vi "Launch Test Bench.vi"(4 "Monitor":enum16{"Primary", "1", "2", "3"}(ring), 6 "Station":T1(ring), 7 "wait until completion? (F)":bool, 8 "error in (no error)":errorcluster, 11 "App Path":path) -> (0 "error out":errorcluster)   [LabVIEW 2019, in "Test Bench Tools.lvlib"]
uses:
  Test Bench Tools.lvlib
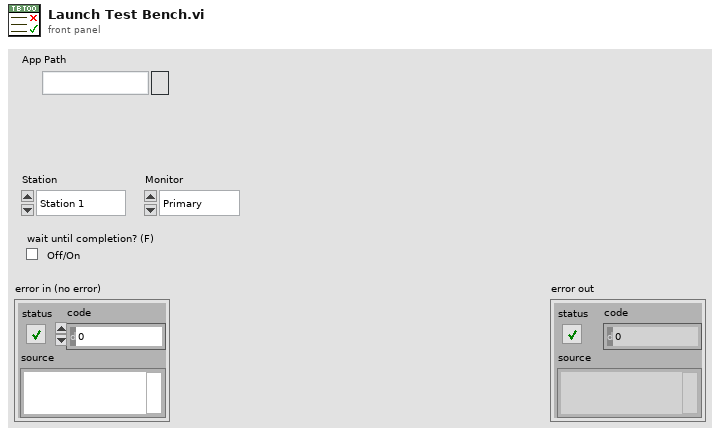
[diagram p1: front panel]
types:
  T1 = enum16{"Station 1", "Station 2", "Station 3", "Station 4"}
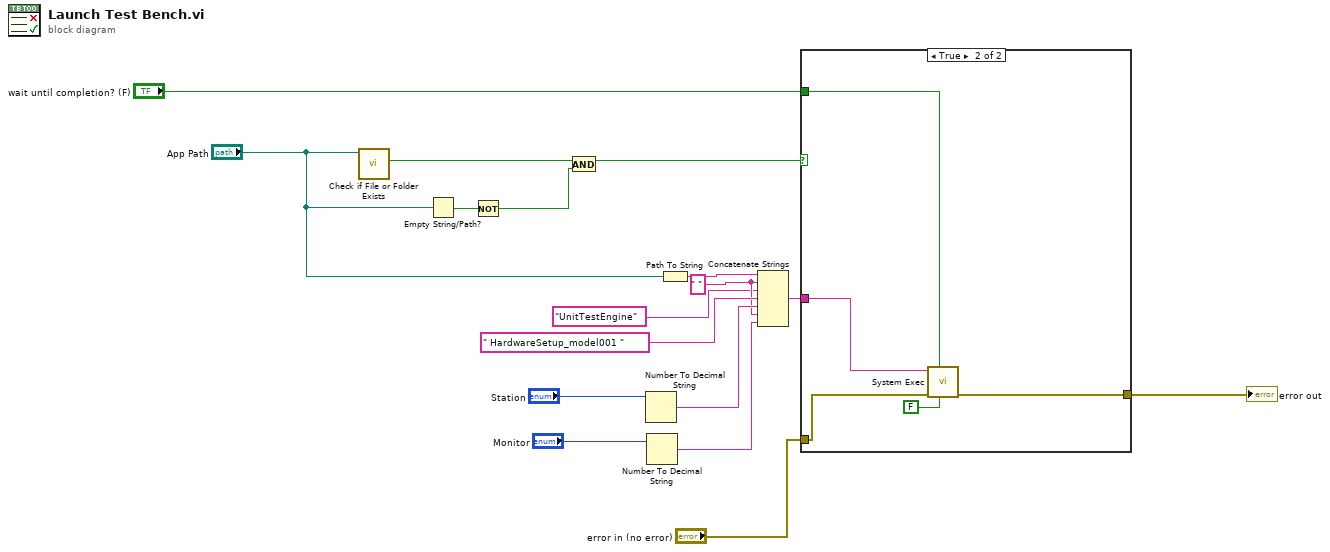
[diagram p0: block diagram]
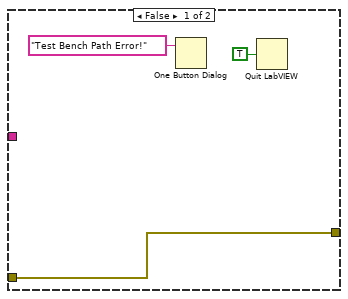
[diagram p2: hidden frame]
diagram:
  w7 = " " ("string")
  n1 = call <vilib>:"Check if File or Folder Exists.vi"("path"="App Path") -> ("file or folder exists?"=w6:bool)  [unwired: 8 in, 2 out]
  n2 = Empty String/Path?(string/path="App Path") -> (empty?=w4:bool)
  n3 = Not(x=w4) -> (.not. x?=w2:bool)
  n4 = And(x=w6, y=w2) -> (x .and. y?=w3:bool)
  n5 = Number To Decimal String(number="Station") -> (decimal integer string=w11:string)  [unwired: 1 in]
  n6 = Number To Decimal String(number="Monitor") -> (decimal integer string=w8:string)  [unwired: 1 in]
  n7 = Path To String(path="App Path") -> (string=w14:string)
  n8 = Concatenate Strings(w14, w7, "UnitTestEngine" ("string"), " HardwareSetup_model001 " ("string"), w11, w7, w8) -> (w12:string)
  n9 = case shown="True" w3 {
    tunnel: "wait until completion? (F)" -> [_ w24]
    tunnel: "error in (no error)" -> [w20 w23]
    tunnel: [w20 w22] -> w15
    tunnel: w12 -> [_ w21]
    frame False {
      n10 = One Button Dialog(message="Test Bench Path Error!") -> ()  [unwired: 1 in, 1 out]
      n11 = Quit LabVIEW(quit? (T)=TRUE) -> ()
    }
    frame True {
      n12 = call <vilib>:"System Exec.vi"("run minimized? (F)"=FALSE, "wait until completion? (T)"=w24, "error in (no error)"=w23, "command line"=w21) -> ("error out"=w22:errorcluster)  [unwired: 4 in, 3 out]
    }
  }
  "error out" <- w15
